vi "Sequencer.vi"() -> ()   [LabVIEW 2013]
uses:
  Tools/vars.ctl
  Tools/Line.ctl
  <vilib>/addons/h5labview2/file/H5Fmode.ctl
  Global.vi
  <vilib>/addons/h5labview2/base/lib_path.vi
  <vilib>/addons/h5labview2/base/H5Equery.vi
  <vilib>/addons/h5labview2/attrib/H5Awrite.llb/H5Awrite.xnode
  <vilib>/addons/h5labview2/file/H5F.lvlib
  <vilib>/addons/h5labview2/group/H5G.lvlib
  <vilib>/addons/h5labview2/attrib/H5A.lvlib
panel:
  in  "SQUID Comment":string
  out "uFiles":path[](array[path])
  in  "Save":bool=TRUE
  in  "stop":bool
  in  "Tab Control":enum32{"Run", "Settings", "Vars"}(tab)
  out "Status":string="<<Idle>>"
  out "Run List":string
  in  "Loops":i32=1 min=1
  in  "Run":bool
  in  "Run Tab":enum32{"Sequencer", "History"}(tab)
  in  "SEQ File":path caption="SEQ File (*.osq)"
  in  "Load List":bool
  out "VAR string":string[](array[string])
  out "Lines":i32
  out "History":cluster{"timestamp":timestamp, "File":path}[](array[cluster])=[{"timestamp"=timestamp(3546777743.6154723 s since 1904-01-01), "File"=path "C:/Users/Adam/Documents/oskar/Examples/example_chan.osq"}]
  out "RID":string="20160522_170223"
  in  "Abort":bool
  in  "Acquire (s)":i32=30
  out "Elapsed (s)":i32=30
  in  "Shuffle":bool
  out "HDF5 Save":path[](array[path])=[path "D:/Data/2016/05/22/20160522_170223/20160522_170223_raw.h5"]
  in  "Save Base":path[](array[path])=[path "D:/Data"]
  in  "Clear Run List Each Run":bool=TRUE
  out "error out":errorcluster
  out "hdf5":errorcluster
  in  "VARS":T1=[{"VAR"="CHAN", "Options"="A", "Val"="1", "Recieved"=FALSE, "Set"=FALSE}, {"VAR"="CHAN", "Options"="B", "Val"="2", "Recieved"=FALSE, "Set"=FALSE}, {"VAR"="CHAN", "Options"="C", "Val"="2", "Recieved"=FALSE, "Set"=FALSE}]
  in  "Override":bool
  out "All Set":bool
  out "Send":bool
  out "Recieved":bool
  in  "Pause":bool caption="Temporary wait before \nsetting next VAR array"
  # "Sequencer"
  # "name"
  # "options"
  # "value"
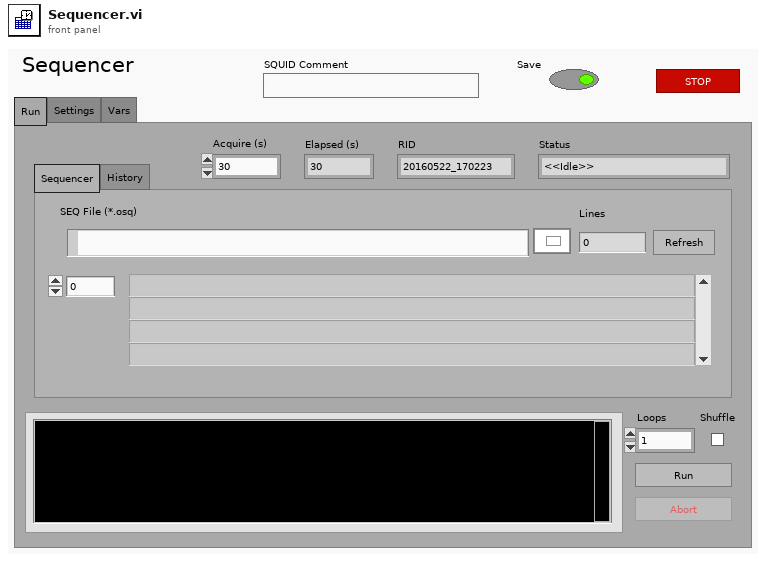
[diagram p1: front panel]
types:
  T1 = typedef "vars.ctl" = cluster{"VAR":string, "Options":string, "Val":string, "Recieved":bool, "Set":bool}[]
  T2 = cluster{"seconds since 1Jan1904":timestamp, string}
  T3 = enum32{"Invalid", "Standard", "Closed", "Hidden", "Minimized", "Maximized"}
  T4 = enum8{"Enabled", "Disabled", "Disabled and Grayed Out"}
  T5 = typedef "Line.ctl" = cluster{"Var Array":string[][], "Comment":string}
  T6 = typedef "H5F.lvlib/H5Fmode.ctl" = enum16{"read-only", "read-write", "overwrite", "create new", "open or create"}
  T7 = cluster{"VAR":string, "Options":string, "Val":string, "Recieved":bool, "Set":bool}
  T8 = cluster{"seconds since 1Jan1904":timestamp, "SEQ File":path}
  T9 = typedef "Semaphore RefNum" = refnum<k1>
  T10 = typedef "hid_t.ctl" = i32
  T11 = cluster{"VAR":string, "Options":string, "Val":string, "Recieved":bool, "Set":bool}[]
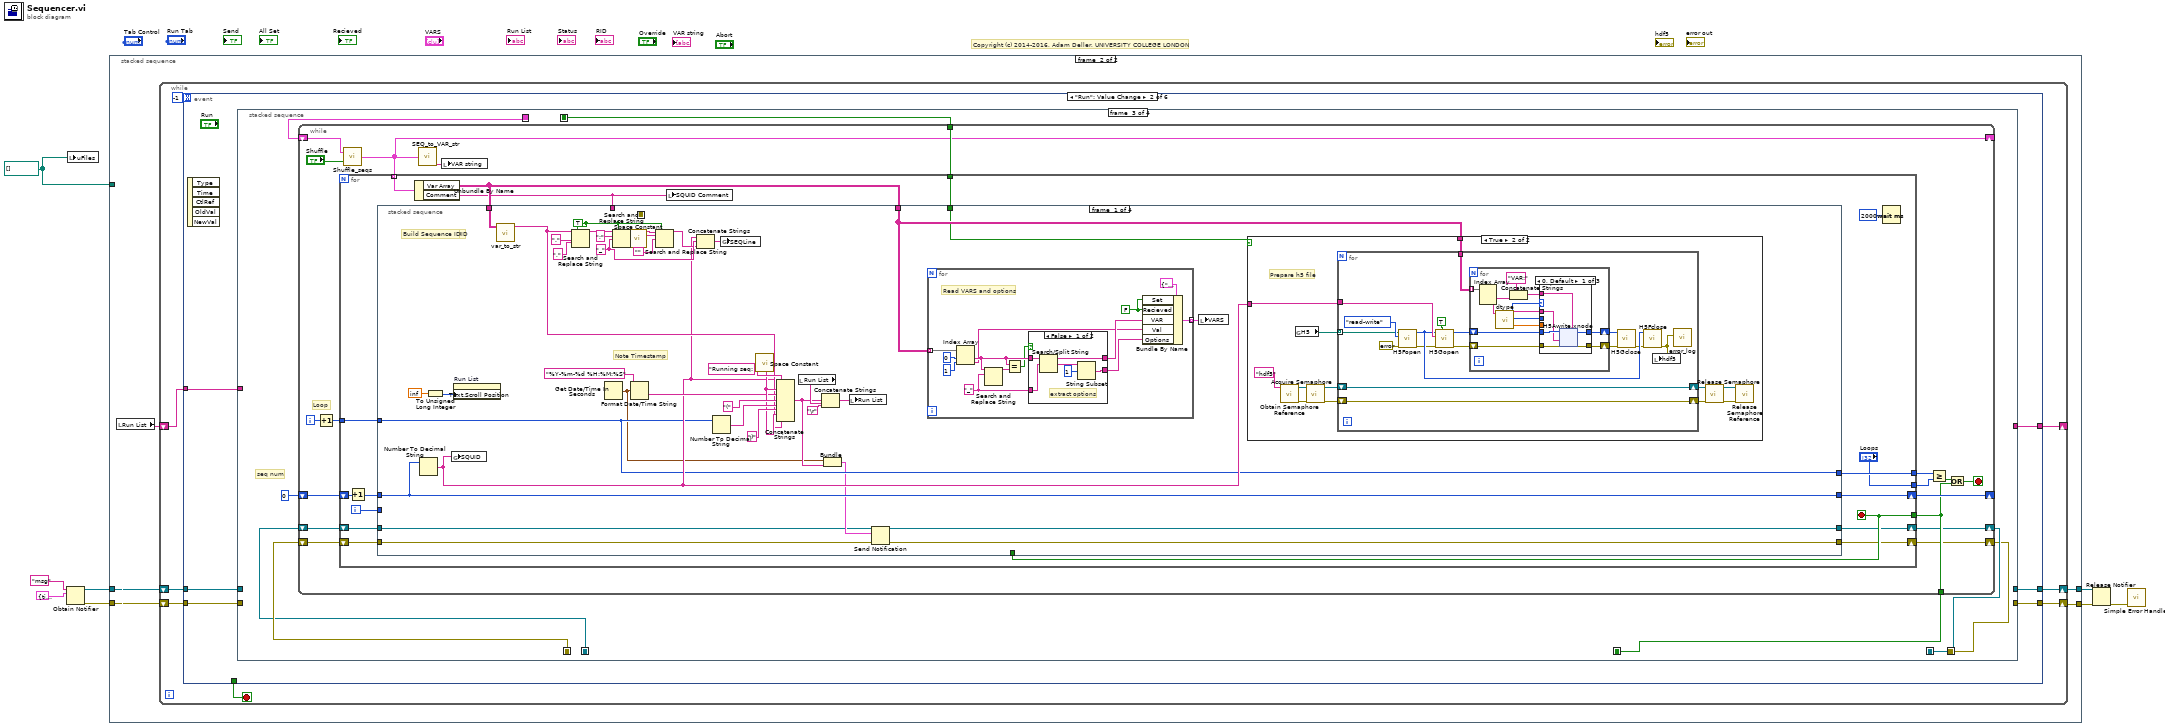
[diagram p0: block diagram]
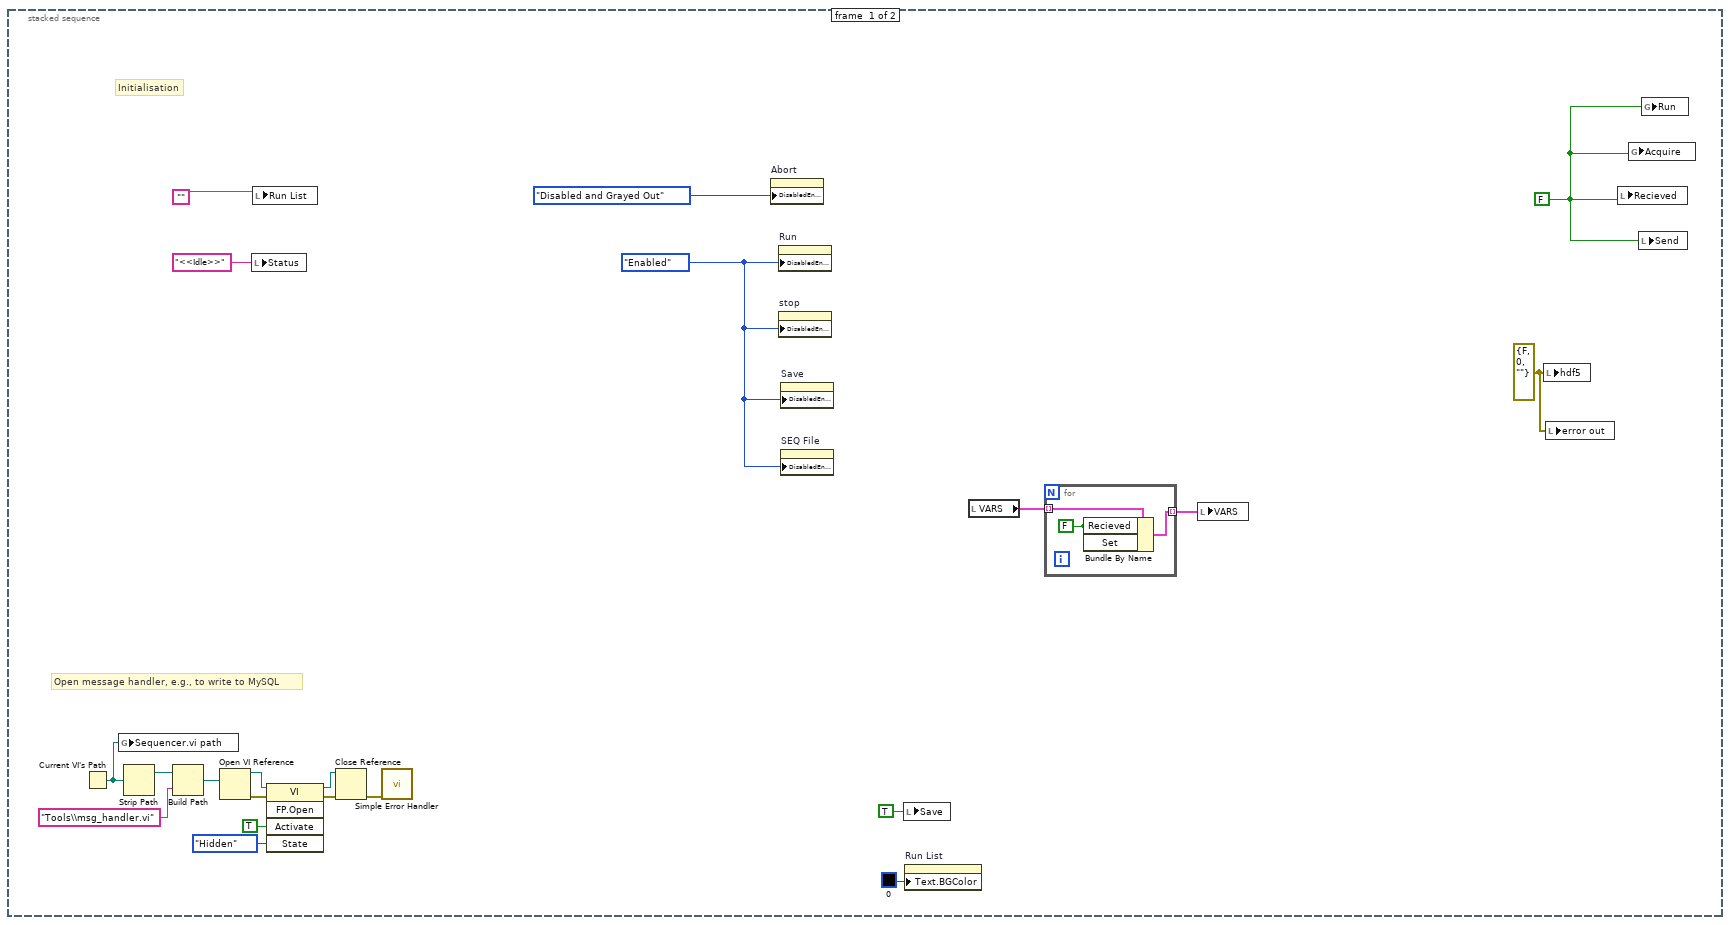
[diagram p2: hidden frame]
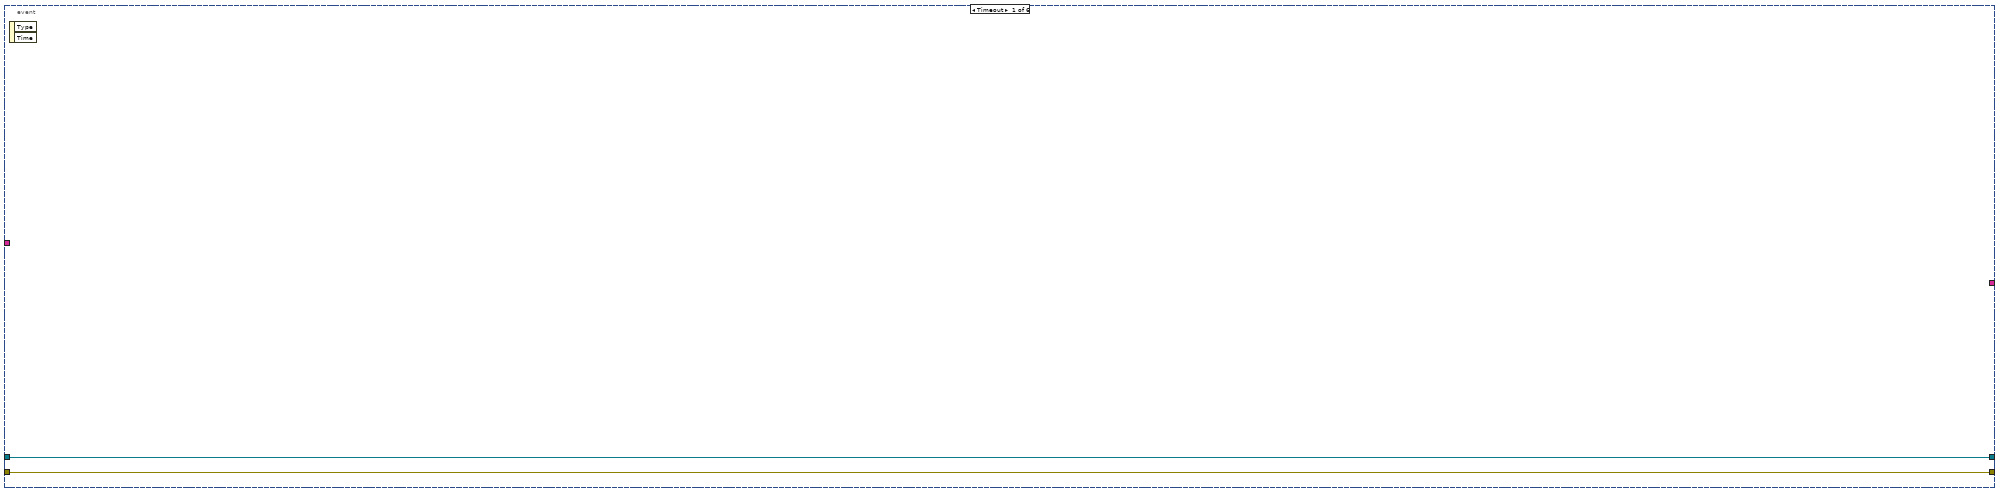
[diagram p3: hidden frame]
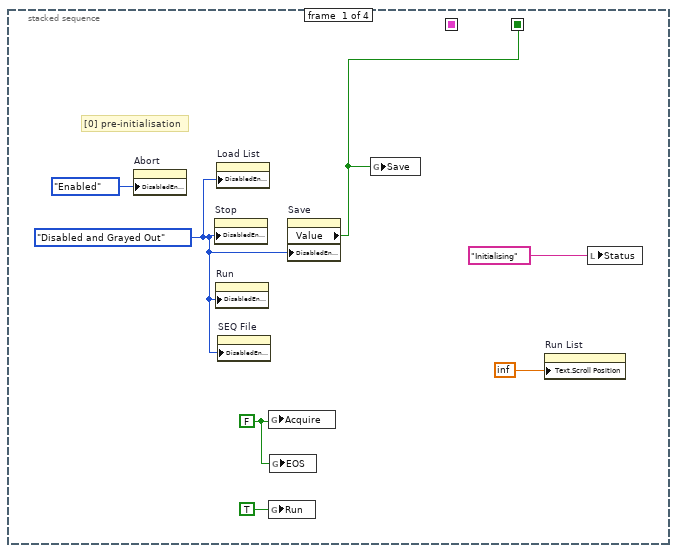
[diagram p4: hidden frame]
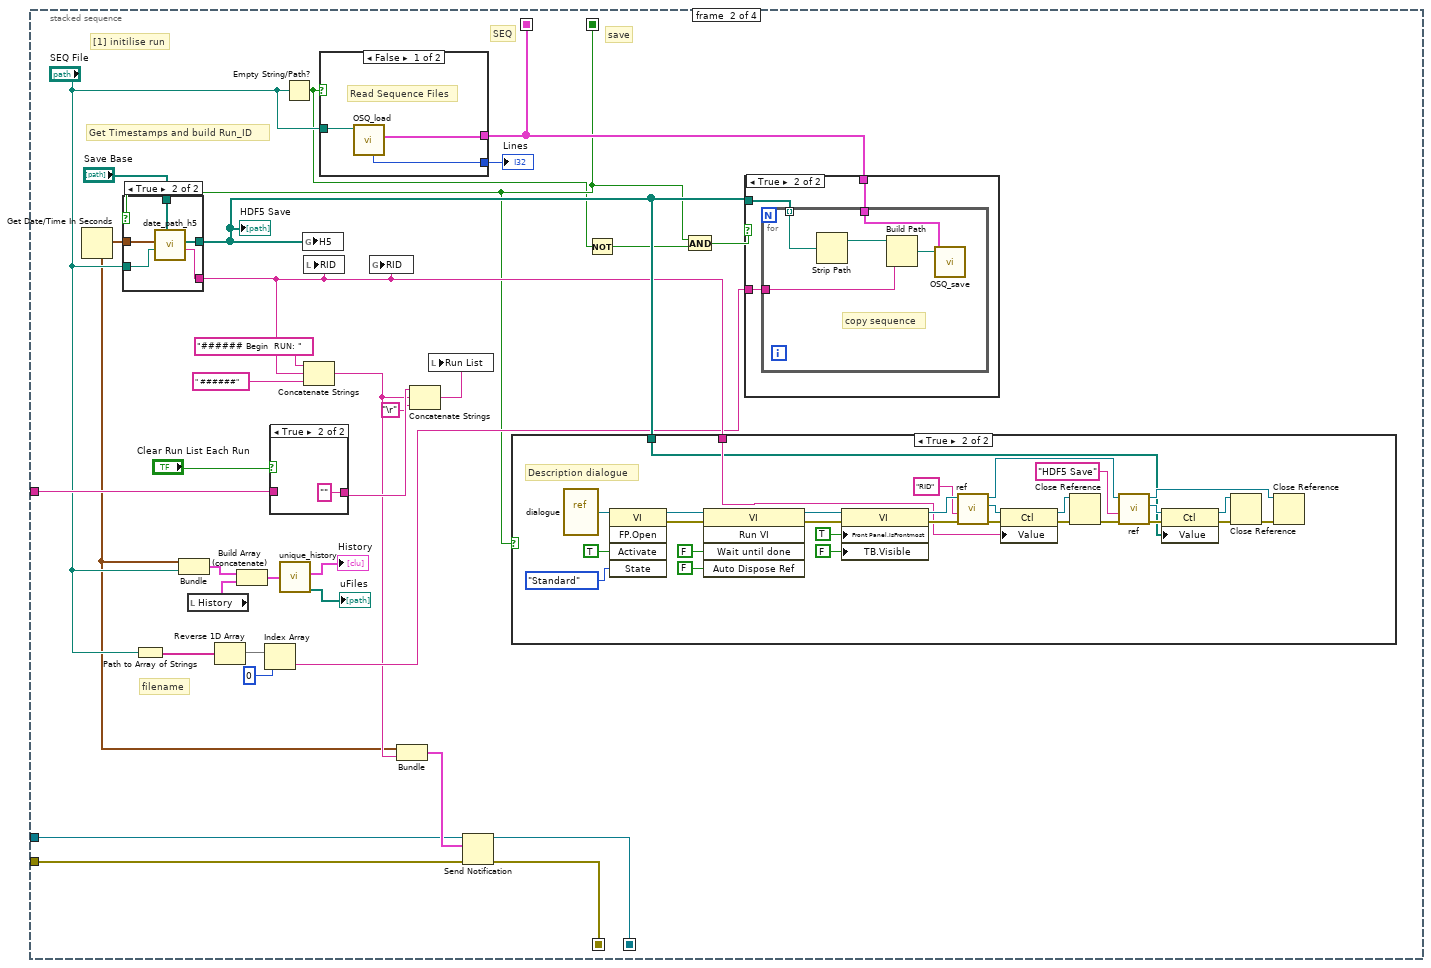
[diagram p5: hidden frame]
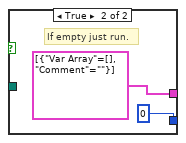
[diagram p7: hidden frame]
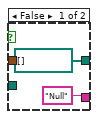
[diagram p8: hidden frame]
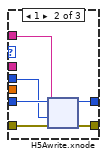
[diagram p12: hidden frame]
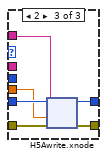
[diagram p13: hidden frame]
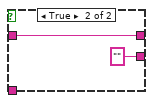
[diagram p14: hidden frame]
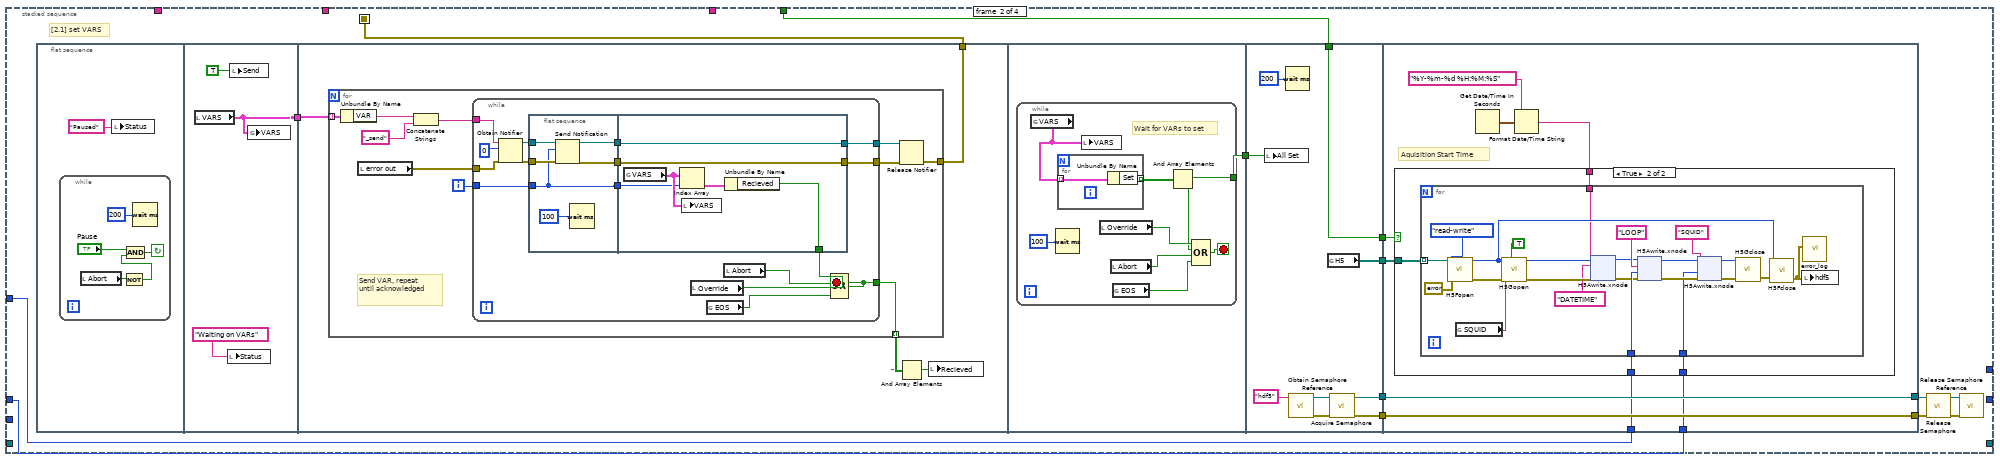
[diagram p15: hidden frame]
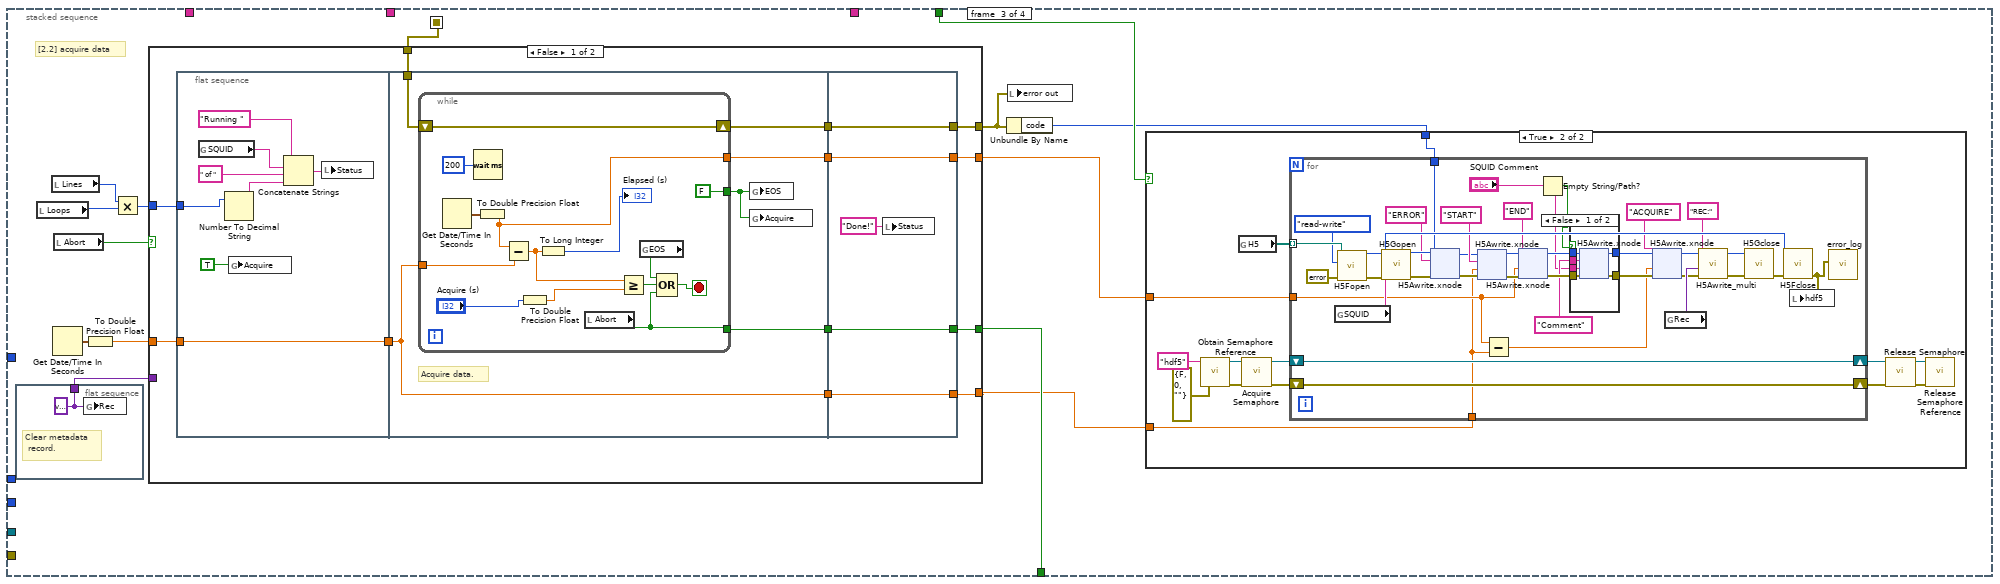
[diagram p17: hidden frame]
diagram:
  w8 = path[] [] ("uFiles")
  # "Copyright (c) 2014-2016, Adam Deller, UNIVERSITY COLLEGE LONDON"
  n1 = Obtain Notifier(name (unnamed)="msg", notification data type=T2 {"seconds since 1Jan1904"=timestamp(0 s since 1904-01-01), ""} ("output cluster")) -> (notifier out=w4:refnum<notifier>, error out=w5:errorcluster)  [unwired: 2 in, 1 out]
  n2 = local write "uFiles"(w8) -> ()
  n3 = stacked-sequence {
    tunnel: w8 -> [_ _]
    tunnel: w4 -> [_ w36]
    tunnel: w5 -> [_ w35]
    tunnel: [_ w34] -> w3
    tunnel: [_ w33] -> w2
    frame #0 {
      w20 = errorcluster {"status"=FALSE, "code"=0, "source"=""} ("hdf5")
      w22 = FALSE ("Send")
      w21 = T4."Enabled" ("Disabled")
      # "Open message handler, e.g., to write to MySQL"
      # "Initialisation"
      n4 = Current VI's Path() -> (path=w19:path)
      n5 = global write "Global.vi" "Sequencer.vi path"(w19) -> ()
      n6 = Strip Path(path=w19) -> (stripped path=w18:path)  [unwired: 1 out]
      n7 = Build Path(base path=w18, name or relative path="Tools\\msg_handler.vi") -> (appended path=w16:path)
      n8 = Open VI Reference(vi path=w16) -> (vi reference=w15:refnum<vi>, error out=w14:errorcluster)  [unwired: 5 in]
      n9 = local write "Status"("<<Idle>>" ("Status")) -> ()
      n10 = local write "Run List"("") -> ()
      n11 = invoke class="VI" method="FP.Open"(reference=w15, error in=w14, "Activate"=TRUE ("Activate?"), "State"=T3."Hidden") -> (reference out=w12:refnum<vi>, error out=w13:errorcluster)  [unwired: 1 in, 3 out]
      n12 = Close Reference(reference=w12, error in (no error)=w13) -> (error out=w9:errorcluster)
      n13 = call <vilib>:"Simple Error Handler.vi"("error in (no error)"=w9) -> ()  [unwired: 4 in, 5 out]
      n14 = property on="Abort" class="Bool (strict)"("DisabledEnum"=T4."Disabled and Grayed Out" ("Disabled")) -> ()  [unwired: 2 in, 2 out]
      n15 = property on="Run" class="Bool"("DisabledEnum"=w21) -> ()  [unwired: 2 in, 2 out]
      n16 = property on="stop" class="Bool"("DisabledEnum"=w21) -> ()  [unwired: 2 in, 2 out]
      n17 = property on="Save" class="Bool (strict)"("DisabledEnum"=w21) -> ()  [unwired: 2 in, 2 out]
      n18 = property on="SEQ File" class="Path"("DisabledEnum"=w21) -> ()  [unwired: 2 in, 2 out]
      n19 = local write "Save"(TRUE ("Save")) -> ()
      n20 = property on="Run List" class="Str"("Text.BGColor"=u32 0) -> ()  [unwired: 2 in, 2 out]
      n21 = local read "VARS"() -> (w27:T1)
      n22 = for {
        tunnel: [w32] -> w26 mode=indexing
        tunnel: w27 -> [w31] mode=indexing
        w30 = FALSE ("Set")
        n23 = Bundle By Name(cluster=w31, "Recieved"=w30, "Set"=w30) -> (w32:T7)
      }
      n24 = local write "VARS"(w26) -> ()
      n25 = local write "hdf5"(w20) -> ()
      n26 = local write "error out"(w20) -> ()
      n27 = local write "Recieved"(w22) -> ()
      n28 = global write "Global.vi" "Acquire"(w22) -> ()
      n29 = local write "Send"(w22) -> ()
      n30 = global write "Global.vi" "Run"(w22) -> ()
    }
    frame #1 {
      n31 = local read "Run List"() -> (w37:string)
      n32 = while {
        shift-right: [w42] -> _
        shift-left: w37 -> [w43]
        shift-right: [w39] -> w33
        shift-left: w36 -> [w41]
        shift-right: [w38] -> w34
        shift-left: w35 -> [w40]
        stop <- w45 stop-if-true
        n33 = event shown="[1] \"Run\": Value Change" {
          selector: _ -> [_ _ _ _ _ _]
          dyn-events: _ -> [_ _ _ _ _ _]
          timeout: -1 -> [_ _ _ _ _ _]
          tunnel: [_ _ _ _ _ "stop"] -> w45
          tunnel: w43 -> [_ w53 _ _ _ _]
          tunnel: [_ w52 _ _ _ _] -> w42
          tunnel: w41 -> [w47 w51 w779 w791 w797 w809]
          tunnel: w40 -> [w46 w50 w778 w790 w796 w808]
          tunnel: [w47 w49 w779 w791 w797 w809] -> w39
          tunnel: [w46 w48 w778 w790 w796 w808] -> w38
          event Timeout {
            n34 = event-data() -> ()  [unwired: 1 in, 2 out]
          }
          event "Run": Value Change {
            n35 = event-data() -> ()  [unwired: 1 in, 5 out]
            n36 = stacked-sequence {
              seq-local: [_ _ w152 _] -> [_ _ _ w760]
              seq-local: [w58 _ _ _] -> [_ w71 w151 _]
              seq-local: [_ w77 _ _] -> [_ _ w149 _]
              seq-local: [_ w62 _ _] -> [_ _ w148 _]
              seq-local: [_ w61 _ _] -> [_ _ w147 _]
              seq-local: [_ _ w146 _] -> [_ _ _ w758]
              seq-local: [_ _ w145 _] -> [_ _ _ w759]
              tunnel: w53 -> [_ w93 _ _]
              tunnel: [_ _ _ w761] -> w52
              tunnel: w51 -> [_ w63 _ _]
              tunnel: w50 -> [_ w65 _ _]
              tunnel: [_ _ _ w754] -> w49
              tunnel: [_ _ _ w753] -> w48
              frame #0 {
                w56 = FALSE ("Save")
                w55 = T4."Disabled and Grayed Out" ("Disabled")
                # "[0] pre-initialisation"
                n37 = property on="Abort" class="Bool (strict)"("DisabledEnum"=T4."Enabled" ("Disabled")) -> ()  [unwired: 2 in, 2 out]
                n38 = property on="Stop" class="Bool"("DisabledEnum"=w55) -> ()  [unwired: 2 in, 2 out]
                n39 = property on="Run" class="Bool"("DisabledEnum"=w55) -> ()  [unwired: 2 in, 2 out]
                n40 = property on="Load List" class="Bool"("DisabledEnum"=w55) -> ()  [unwired: 2 in, 2 out]
                n41 = property on="SEQ File" class="Path"("DisabledEnum"=w55) -> ()  [unwired: 2 in, 2 out]
                n42 = global write "Global.vi" "Acquire"(w56) -> ()
                n43 = global write "Global.vi" "Run"(TRUE ("Run on now")) -> ()
                n44 = global write "Global.vi" "EOS"(w56) -> ()
                n45 = property on="Save" class="Bool (strict)"("DisabledEnum"=w55) -> ("Value"=w58:bool)  [unwired: 2 in, 2 out]
                n46 = global write "Global.vi" "Save"(w58) -> ()
                n47 = property on="Run List" class="Str"("Text.Scroll Position"=inf) -> ()  [unwired: 2 in, 2 out]
                n48 = local write "Status"("Initialising" ("Status")) -> ()
              }
              frame #1 {
                # "filename"
                # "save"
                # "SEQ"
                # "[1] initilise run"
                # "Get Timestamps and build Run_ID"
                n49 = Get Date/Time In Seconds() -> (seconds since 1Jan1904=w66:timestamp)
                n50 = case shown="True" w71 {
                  tunnel: w66 -> [_ w134]
                  tunnel: ["Null" ("RID") w133] -> w78
                  tunnel: "Save Base" -> [_ w132]
                  tunnel: [path[] [] ("Paths") w131] -> w79
                  tunnel: "SEQ File" -> [_ w130]
                  frame False {
                  }
                  frame True {
                    n51 = call "date_path_h5.vi"("Bases"=w132, "SEQ File"=w130, "time stamp"=w134) -> ("RID"=w133:string, "H5"=w131:path[])  [unwired: 7 in]
                  }
                }
                "HDF5 Save" <- w79
                n52 = Path to Array of Strings(0:"SEQ File") -> (2:w75:string[])  [unwired: 1 out]
                n53 = Bundle("seconds since 1Jan1904"=w66, "SEQ File"="SEQ File") -> (w81:T8)  [unwired: 1 in]
                n54 = local read "History"() -> (w85:cluster{"timestamp":timestamp, "File":path}[])
                n55 = Reverse 1D Array(array=w75) -> (reversed array=w74:string[])
                n56 = Build Array (concatenate)(w81, w85) -> (w84:cluster{"timestamp":timestamp, "File":path}[])
                n57 = Index Array(array=w74, index=0) -> (element=w72:string)
                n58 = case shown="True" "Clear Run List Each Run" {
                  tunnel: w93 -> [w143 _]
                  tunnel: [w143 "" ("Log")] -> w91
                  frame False {
                  }
                  frame True {
                  }
                }
                n59 = call "unique_history.vi"("History In"=w84) -> ("uFiles"=→"uFiles":path[], "History Out"=→"History":cluster{"Time Stamp":timestamp, "Path":path}[])  [unwired: 9 in]
                n60 = Empty String/Path?(string/path="SEQ File") -> (empty?=w70:bool)
                n61 = global write "Global.vi" "H5"(w79) -> ()
                n62 = local write "RID"(w78) -> ()
                n63 = Concatenate Strings("###### Begin  RUN: " ("string"), w78, " ######" ("string")) -> (w67:string)
                n64 = case shown="False" w70 {
                  tunnel: "SEQ File" -> [w124 _]
                  tunnel: [w125 0 ("Lines")] -> w80
                  tunnel: [w123 T5[] [{"Var Array"=[], "Comment"=""}] ("SEQs")] -> w77
                  frame False {
                    # "Read Sequence Files"
                    n65 = call "OSQ_load.vi"("Open"=w124) -> ("SEQs"=w123:T5[], "Lines"=w125:i32)  [unwired: 7 in, 2 out]
                  }
                  frame True {
                    # "If empty just run."
                  }
                }
                "Lines" <- w80
                n66 = global write "Global.vi" "RID"(w78) -> ()
                n67 = Bundle("seconds since 1Jan1904"=w66, w67) -> (w64:T2)  [unwired: 1 in]
                n68 = Concatenate Strings(w91, w67, "\r") -> (w90:string)
                n69 = local write "Run List"(w90) -> ()
                n70 = Send Notification(notification=w64, notifier=w63, error in (no error)=w65) -> (notifier out=w61:refnum<notifier>, error out=w62:errorcluster)
                n71 = case shown="True" w71 {
                  tunnel: w79 -> [_ w94]
                  tunnel: w78 -> [_ w95]
                  frame False {
                  }
                  frame True {
                    # "Description dialogue"
                    n72 = vi-ref "dialogue.vi"() -> (w121:refnum<vi>)
                    n73 = invoke class="VI" method="FP.Open"(reference=w121, "Activate"=TRUE ("Activate?"), "State"=T3."Standard") -> (reference out=w102:refnum<vi>, error out=w99:errorcluster)  [unwired: 2 in, 3 out]
                    n74 = invoke class="VI" method="Run VI"(reference=w102, error in=w99, "Wait until done"=FALSE ("Wait Until Done"), "Auto Dispose Ref"=FALSE ("Auto Dispose Reference")) -> (reference out=w101:refnum<vi>, error out=w100:errorcluster)  [unwired: 1 in, 3 out]
                    n75 = property class="VI"(reference=w101, error in=w100, "Front Panel.IsFrontmost"=TRUE ("Front Panel Window:Is Frontmost"), "TB.Visible"=FALSE ("Tool Bar:Visible")) -> (reference out=w118:refnum<vi>, error out=w117:errorcluster)
                    n76 = call "ref.vi"("error in (no error)"=w117, "Name"="RID", "VI reference"=w118) -> ("error out"=w111:errorcluster, "Ctrl reference out"=w112:refnum<vi>, "VI reference out"=w115:refnum<vi>)  [unwired: 5 in, 1 out]
                    n77 = property class="Ctl"(reference=w112, error in=w111, "Value"=w95) -> (reference out=w109:refnum<vi>, error out=w110:errorcluster)
                    n78 = Close Reference(reference=w109, error in (no error)=w110) -> (error out=w108:errorcluster)
                    n79 = call "ref.vi"("error in (no error)"=w108, "Name"="HDF5 Save", "VI reference"=w115) -> ("error out"=w107:errorcluster, "Ctrl reference out"=w103:refnum<vi>, "VI reference out"=w113:refnum<vi>)  [unwired: 5 in, 1 out]
                    n80 = property class="Ctl"(reference=w103, error in=w107, "Value"=w94) -> (reference out=w104:refnum<vi>, error out=w106:errorcluster)
                    n81 = Close Reference(reference=w104, error in (no error)=w106) -> (error out=w105:errorcluster)
                    n82 = Close Reference(reference=w113, error in (no error)=w105) -> ()  [unwired: 1 out]
                  }
                }
                n83 = Not(x=w70) -> (.not. x?=w69:bool)
                n84 = And(x=w71, y=w69) -> (x .and. y?=w68:bool)
                n85 = case shown="True" w68 {
                  tunnel: w72 -> [_ w137]
                  tunnel: w79 -> [_ w136]
                  tunnel: w77 -> [_ w135]
                  frame False {
                  }
                  frame True {
                    n86 = for {
                      tunnel: w137 -> [w138]
                      tunnel: w136 -> [w140] mode=indexing
                      tunnel: w135 -> [w141]
                      # "copy sequence"
                      n87 = Strip Path(path=w140) -> (stripped path=w139:path)  [unwired: 1 out]
                      n88 = Build Path(base path=w139, name or relative path=w138) -> (appended path=w142:path)
                      n89 = call "OSQ_save.vi"("SEQs"=w141, "Save"=w142) -> ()  [unwired: 8 in, 2 out]
                    }
                  }
                }
              }
              frame #2 {
                # "seq num"
                n90 = while {
                  tunnel: [w157] -> w152
                  tunnel: w151 -> [w170]
                  shift-right: [w168] -> _
                  shift-left: 0 -> [w169]
                  shift-right: [w162] -> _
                  shift-left: w149 -> [w164]
                  shift-right: [w153] -> w146
                  shift-left: w147 -> [w156]
                  shift-right: [w154] -> w145
                  shift-left: w148 -> [w155]
                  i -> [w166]
                  stop <- w159 stop-if-true
                  # "Loop"
                  n91 = Increment(x=w166) -> (x+1=w167:i32)
                  n92 = call "Shuffle_seqs.vi"("Shuffle"="Shuffle", "Array IN"=w164) -> ("Array OUT"=w162:T5[])
                  n93 = for {
                    tunnel: [w175] -> w157
                    tunnel: w170 -> [w187]
                    shift-right: [w185] -> w168
                    shift-left: w169 -> [w181]
                    tunnel: w162 -> [w183] mode=indexing
                    tunnel: w167 -> [w180]
                    tunnel: [w177] -> w161
                    tunnel: ["Loops"] -> w158
                    shift-right: [w172] -> w153
                    shift-left: w156 -> [w174]
                    shift-right: [w171] -> w154
                    shift-left: w155 -> [w173]
                    i -> [w184]
                    stop <- w175 stop-if-true
                    n94 = Increment(x=w181) -> (x+1=w182:i32)
                    n95 = Unbundle By Name(w183) -> ("Var Array"=w179:string[][], "Comment"=w178:string)
                    n96 = stacked-sequence {
                      seq-local: [_ w372 _ _] -> [_ _ w548 _]
                      tunnel: [_ _ w547 _] -> w175
                      tunnel: w187 -> [w198 w363 w545 _]
                      tunnel: [w215 _ _ _] -> w185
                      tunnel: w184 -> [_ _ _ _]
                      tunnel: w179 -> [w199 _ _ _]
                      tunnel: w182 -> [w215 w360 _ _]
                      tunnel: w180 -> [w196 w361 _ _]
                      tunnel: w178 -> [_ _ _ _]
                      tunnel: w179 -> [w201 _ _ _]
                      tunnel: [w196 _ _ _] -> w177
                      tunnel: w174 -> [w191 _ _ _]
                      tunnel: w173 -> [w190 _ _ _]
                      tunnel: [w189 _ _ _] -> w172
                      tunnel: [w188 _ _ _] -> w171
                      frame #0 {
                        w207 = TRUE ("replace all? (F)")
                        w206 = "_" ("replace string (\"\")")
                        # "[2.0] initialise SQUID"
                        # "Note Timestamp"
                        # "Build Sequence ID"
                        n97 = Number To Decimal String(number=w215) -> (decimal integer string=w197:string)  [unwired: 1 in]
                        n98 = To Unsigned Long Integer(number=inf) -> (unsigned 32bit integer=w202:u32)
                        n99 = global write "Global.vi" "SQUID"(w197) -> ()
                        n100 = property on="Run List" class="Str"("Text.Scroll Position"=w202) -> ()  [unwired: 2 in, 2 out]
                        n101 = call "var_to_str.vi"("Var Array"=w201) -> ("VAR string"=w200:string)  [unwired: 10 in]
                        n102 = Search and Replace String(replace all?=w207, input string=w200, search string=".", replace string="," ("replace string (\"\")")) -> (result string=w208:string)  [unwired: 4 in, 3 out]
                        n103 = Get Date/Time In Seconds() -> (seconds since 1Jan1904=w193:timestamp)
                        n104 = Search and Replace String(replace all?=w207, input string=w208, search string=";", replace string=w206) -> (result string=w211:string)  [unwired: 4 in, 3 out]
                        n105 = call <vilib>:"Space Constant.vi"() -> ("String"=w213:string)
                        n106 = Format Date/Time String(time format string (%c)="%Y-%m-%d %H:%M:%S", seconds (now)=w193) -> (date/time string=w219:string)  [unwired: 1 in]
                        n107 = Search and Replace String(replace all?=w207, input string=w211, search string=w213, replace string="") -> (result string=w205:string)  [unwired: 4 in, 3 out]
                        n108 = Concatenate Strings(w197, w206, w205) -> (w204:string)
                        n109 = Number To Decimal String(number=w196) -> (decimal integer string=w222:string)  [unwired: 1 in]
                        n110 = global write "Global.vi" "SEQLine"(w204) -> ()
                        n111 = call <vilib>:"Space Constant.vi"() -> ("String"=w220:string)
                        n112 = Concatenate Strings(w219, w220, "Running seq: " ("string"), w197, "(" ("string"), w222, ")" ("string"), w220, w200) -> (w194:string)
                        n113 = local read "Run List"() -> (w218:string)
                        n114 = Concatenate Strings(w218, w194, "\r") -> (w217:string)
                        n115 = Bundle("seconds since 1Jan1904"=w193, w194) -> (w192:T2)  [unwired: 1 in]
                        n116 = local write "Run List"(w217) -> ()
                        n117 = Send Notification(notification=w192, notifier=w191, error in (no error)=w190) -> (notifier out=w189:refnum<notifier>, error out=w188:errorcluster)
                        n118 = for {
                          tunnel: w199 -> [w349] mode=indexing
                          tunnel: [w348] -> w195 mode=indexing
                          w341 = "_" ("search string/char (-)")
                          w346 = FALSE ("Set")
                          # "Read VARS and options"
                          n119 = Index Array(array=w349, index #1=0 ("index"), index #2=1 ("index")) -> (element #1=w342:string, element #2=w339:string)
                          n120 = Search and Replace String(input string=w342, search string=w341) -> (result string=w343:string)  [unwired: 6 in, 3 out]
                          n121 = Equal?(x=w342, y=w343) -> (x = y?=w340:bool)
                          n122 = case shown="False" w340 {
                            tunnel: [w357 w358] -> w345
                            tunnel: [w354 "" ("String")] -> w344
                            tunnel: w342 -> [w353 w358]
                            tunnel: w341 -> [w352 _]
                            frame False {
                              # "extract options"
                              n123 = Search/Split String(string=w353, search string/char (-)=w352) -> (substring before match=w357:string, match + rest of string=w356:string)  [unwired: 1 in, 1 out]
                              n124 = String Subset(string=w356, offset (0)=1) -> (substring=w354:string)  [unwired: 1 in]
                            }
                            frame True {
                            }
                          }
                          n125 = Bundle By Name(cluster=T7 {"VAR"="", "Options"="", "Val"="", "Recieved"=FALSE, "Set"=FALSE} ("VARS 2"), "Set"=w346, "Recieved"=w346, "VAR"=w345, "Val"=w339, "Options"=w344) -> (w348:T7)
                        }
                        n126 = local write "VARS"(w195) -> ()
                        n127 = case shown="True" w198 {
                          tunnel: w197 -> [_ w236]
                          tunnel: w199 -> [_ w235]
                          frame False {
                          }
                          frame True {
                            # "Prepare h5 file"
                            n128 = call <vilib>:"Obtain Semaphore Reference.vi"("name (unnamed)"="hdf5") -> ("error out"=w233:errorcluster, "semaphore"=w234:T9)  [unwired: 4 in, 1 out]
                            n129 = global read "Global.vi" "H5"() -> (w237:path[])
                            n130 = call <vilib>:"Acquire Semaphore.vi"("error in (no error)"=w233, "semaphore"=w234) -> ("error out"=w228:errorcluster, "semaphore out"=w229:T9)  [unwired: 3 in, 1 out]
                            n131 = for {
                              tunnel: w237 -> [w252] mode=indexing
                              tunnel: w236 -> [w251]
                              tunnel: w235 -> [w245]
                              shift-right: [w243] -> w227
                              shift-left: w229 -> [w243]
                              shift-right: [w244] -> w226
                              shift-left: w228 -> [w244]
                              n132 = call <vilib>:"H5Fopen.vi"("error in (no error)"=errorcluster {"status"=FALSE, "code"=0, "source"=""} ("error out"), "mode (read-only)"=H5Fmode."read-write", "path"=w252) -> ("error out"=w242:errorcluster, "ref out"=w249:T10)  [unwired: 7 in]
                              n133 = call <vilib>:"H5Gopen.vi"("create? (F)"=TRUE, "error in (no error)"=w242, "name"=w251, "ref in"=w249) -> ("error out"=w241:errorcluster, "group out"=w240:T10)  [unwired: 6 in]
                              n134 = for {
                                tunnel: w245 -> [w264] mode=indexing
                                shift-right: [w266] -> w247
                                shift-left: w240 -> [w259]
                                shift-right: [w265] -> w246
                                shift-left: w241 -> [w258]
                                n135 = Index Array(array=w264) -> (element #1=w263:string, element #2=w260:string)  [unwired: 2 in]
                                n136 = call "dtype.vi"("String"=w260) -> ("DBL"=w254:dbl, "I32"=w255:i32, "String out"=w256:string, "dtype (0:str, 1:i32, 2:f64)"=w257:u32)  [unwired: 7 in]
                                n137 = Concatenate Strings("VAR:" ("string"), w263) -> (w261:string)
                                n138 = case shown="0, Default" w257 {
                                tunnel: [w270 w296 w318] -> w266
                                tunnel: [w271 w295 w319] -> w265
                                tunnel: w261 -> [w268 w294 w316]
                                tunnel: w259 -> [w269 w293 w317]
                                tunnel: w258 -> [w272 w292 w320]
                                tunnel: w256 -> [w267 _ _]
                                tunnel: w255 -> [_ w291 _]
                                tunnel: w254 -> [_ _ w315]
                                frame 0, Default {
                                n139 = xnode "H5Awrite.xnode"("error in (no error)"=w272, "data"=w267, "attrib name"=w268, "ref in"=w269) -> ("error out"=w271:errorcluster, "ref out"=w270:i32)  [unwired: 3 in, 1 out]
                                }
                                frame 1 {
                                n140 = xnode "H5Awrite.xnode"("error in (no error)"=w292, "data"=w291, "attrib name"=w294, "ref in"=w293) -> ("error out"=w295:errorcluster, "ref out"=w296:i32)  [unwired: 3 in, 1 out]
                                }
                                frame 2 {
                                n141 = xnode "H5Awrite.xnode"("error in (no error)"=w320, "data"=w315, "attrib name"=w316, "ref in"=w317) -> ("error out"=w319:errorcluster, "ref out"=w318:i32)  [unwired: 3 in, 1 out]
                                }
                                }
                              }
                              n142 = call <vilib>:"H5Gclose.vi"("error in (no error)"=w246, "group in"=w247) -> ("error out"=w248:errorcluster)  [unwired: 9 in]
                              n143 = call <vilib>:"H5Fclose.vi"("error in (no error)"=w248, "ref"=w249) -> ("error out"=w238:errorcluster)  [unwired: 9 in]
                              n144 = local write "hdf5"(w238) -> ()
                              n145 = call "error_log.vi"("error"=w238) -> ()  [unwired: 10 in]
                            }
                            n146 = call <vilib>:"Release Semaphore.vi"("error in (no error)"=w226, "semaphore"=w227) -> ("error out"=w231:errorcluster, "semaphore out"=w230:T9)  [unwired: 4 in]
                            n147 = call <vilib>:"Release Semaphore Reference.vi"("error in (no error)"=w231, "semaphore"=w230) -> ()  [unwired: 8 in, 2 out]
                          }
                        }
                      }
                      frame #1 {
                        # "[2.1] set VARS"
                        n148 = flat-sequence {
                          tunnel: [w382] -> w373
                          tunnel: w373 -> [w386]
                          tunnel: [w383] -> w372
                          tunnel: [w425] -> w371
                          tunnel: w371 -> [w443]
                          tunnel: [w439] -> w367
                          tunnel: [w438] -> w365
                          tunnel: [w437] -> w364
                          tunnel: w363 -> [w437]
                          tunnel: [w436] -> w362
                          tunnel: [w452] -> w368
                          tunnel: w367 -> [w452]
                          tunnel: [w451] -> w366
                          tunnel: w365 -> [w451]
                          tunnel: w364 -> [w450]
                          tunnel: w362 -> [w449]
                          tunnel: w361 -> [w446]
                          tunnel: w360 -> [w445]
                          frame #0 {
                            n149 = while {
                              stop <- w377 continue-if-true
                              n150 = local read "Abort"() -> (w378:bool)
                              n151 = Not(x=w378) -> (.not. x?=w376:bool)
                              n152 = And(x="Pause", y=w376) -> (x .and. y?=w377:bool)
                              n153 = Wait (ms)(milliseconds to wait=u32 200) -> ()  [unwired: 1 out]
                            }
                            n154 = local write "Status"("Paused" ("Status")) -> ()
                          }
                          frame #1 {
                            n155 = local read "VARS"() -> (w382:T1)
                            n156 = local write "Status"("Waiting on VARs" ("Status")) -> ()
                            n157 = local write "Send"(TRUE ("Send")) -> ()
                            n158 = global write "Global.vi" "VARS"(w382) -> ()
                          }
                          frame #2 {
                            n159 = for {
                              tunnel: w386 -> [w396] mode=indexing
                              tunnel: [w392] -> w385 mode=indexing
                              tunnel: [w389] -> w383
                              i -> [w393]
                              # "Send VAR, repeat until acknowledged"
                              n160 = Unbundle By Name(w396) -> ("VAR"=w394:string)
                              n161 = local read "error out"() -> (w387:errorcluster)
                              n162 = Concatenate Strings(w394, "_send") -> (w388:string)
                              n163 = while {
                                tunnel: w393 -> [w408]
                                tunnel: [w403] -> w392
                                tunnel: [w411] -> w391
                                tunnel: [w410] -> w390
                                tunnel: w388 -> [w401]
                                tunnel: w387 -> [w397]
                                stop <- w403 stop-if-true
                                n164 = Obtain Notifier(name (unnamed)=w401, notification data type=0, error in (no error)=w397) -> (notifier out=w399:refnum<notifier>, error out=w400:errorcluster)  [unwired: 1 in, 1 out]
                                n165 = flat-sequence {
                                tunnel: w399 -> [w417]
                                tunnel: w400 -> [w418]
                                tunnel: [w416] -> w412
                                tunnel: [w415] -> w409
                                tunnel: w408 -> [w413]
                                tunnel: [w413] -> w407
                                tunnel: [w421] -> w404
                                tunnel: [w423] -> w411
                                tunnel: w412 -> [w423]
                                tunnel: [w422] -> w410
                                tunnel: w409 -> [w422]
                                tunnel: w407 -> [w419]
                                frame #0 {
                                n166 = Send Notification(notification=w413, notifier=w417, error in (no error)=w418) -> (notifier out=w416:refnum<notifier>, error out=w415:errorcluster)
                                n167 = Wait (ms)(milliseconds to wait=u32 100) -> ()  [unwired: 1 out]
                                }
                                frame #1 {
                                n168 = global read "Global.vi" "VARS"() -> (w420:T11)
                                n169 = Index Array(array=w420, index=w419) -> (element=w424:T7)
                                n170 = local write "VARS"(w420) -> ()
                                n171 = Unbundle By Name(w424) -> ("Recieved"=w421:bool)
                                }
                                }
                                n172 = local read "Override"() -> (w405:bool)
                                n173 = global read "Global.vi" "EOS"() -> (w398:bool)
                                n174 = local read "Abort"() -> (w406:bool)
                                n175 = Compound Arithmetic op=OR(w404, w406, w405, w398) -> (w403:bool)
                              }
                              n176 = Release Notifier(notifier=w391, error in (no error)=w390) -> (error out=w389:errorcluster)  [unwired: 1 in, 2 out]
                            }
                            n177 = And Array Elements(Boolean array=w385) -> (logical AND=w384:bool)
                            n178 = local write "Recieved"(w384) -> ()
                          }
                          frame #3 {
                            n179 = while {
                              tunnel: [w428] -> w425
                              stop <- w427 stop-if-true
                              # "Wait for VARs to set"
                              n180 = global read "Global.vi" "VARS"() -> (w431:T11)
                              n181 = Wait (ms)(milliseconds to wait=u32 100) -> ()  [unwired: 1 out]
                              n182 = for {
                                tunnel: w431 -> [w435] mode=indexing
                                tunnel: [w434] -> w433 mode=indexing
                                n183 = Unbundle By Name(w435) -> ("Set"=w434:bool)
                              }
                              n184 = local write "VARS"(w431) -> ()
                              n185 = local read "Override"() -> (w430:bool)
                              n186 = local read "Abort"() -> (w429:bool)
                              n187 = global read "Global.vi" "EOS"() -> (w426:bool)
                              n188 = And Array Elements(Boolean array=w433) -> (logical AND=w428:bool)
                              n189 = Compound Arithmetic op=OR(w430, w428, w429, w426) -> (w427:bool)
                            }
                          }
                          frame #4 {
                            n190 = local write "All Set"(w443) -> ()
                            n191 = Wait (ms)(milliseconds to wait=u32 200) -> ()  [unwired: 1 out]
                            n192 = call <vilib>:"Obtain Semaphore Reference.vi"("name (unnamed)"="hdf5") -> ("error out"=w441:errorcluster, "semaphore"=w440:T9)  [unwired: 4 in, 1 out]
                            n193 = global read "Global.vi" "H5"() -> (w436:path[])
                            n194 = call <vilib>:"Acquire Semaphore.vi"("error in (no error)"=w441, "semaphore"=w440) -> ("error out"=w438:errorcluster, "semaphore out"=w439:T9)  [unwired: 3 in, 1 out]
                          }
                          frame #5 {
                            # "Aquisition Start Time"
                            n195 = Get Date/Time In Seconds() -> (seconds since 1Jan1904=w447:timestamp)
                            n196 = Format Date/Time String(time format string (%c)="%Y-%m-%d %H:%M:%S", seconds (now)=w447) -> (date/time string=w448:string)  [unwired: 1 in]
                            n197 = case shown="True" w450 {
                              tunnel: w449 -> [_ w457]
                              tunnel: w448 -> [_ w456]
                              tunnel: w446 -> [_ w455]
                              tunnel: w445 -> [_ w454]
                              frame False {
                              }
                              frame True {
                                n198 = for {
                                tunnel: w457 -> [w479] mode=indexing
                                tunnel: w456 -> [w474]
                                tunnel: w455 -> [w468]
                                tunnel: w454 -> [w462]
                                n199 = call <vilib>:"H5Fopen.vi"("error in (no error)"=errorcluster {"status"=FALSE, "code"=0, "source"=""} ("error out"), "mode (read-only)"=H5Fmode."read-write", "path"=w479) -> ("error out"=w477:errorcluster, "ref out"=w476:T10)  [unwired: 7 in]
                                n200 = global read "Global.vi" "SQUID"() -> (w470:string)
                                n201 = call <vilib>:"H5Gopen.vi"("create? (F)"=TRUE, "error in (no error)"=w477, "name"=w470, "ref in"=w476) -> ("error out"=w472:errorcluster, "group out"=w473:T10)  [unwired: 6 in]
                                n202 = xnode "H5Awrite.xnode"("error in (no error)"=w472, "data"=w474, "attrib name"="DATETIME", "ref in"=w473) -> ("error out"=w460:errorcluster, "ref out"=w461:i32)  [unwired: 3 in, 1 out]
                                n203 = xnode "H5Awrite.xnode"("error in (no error)"=w460, "data"=w468, "attrib name"="LOOP", "ref in"=w461) -> ("error out"=w467:errorcluster, "ref out"=w464:i32)  [unwired: 3 in, 1 out]
                                n204 = xnode "H5Awrite.xnode"("error in (no error)"=w467, "data"=w462, "attrib name"="SQUID", "ref in"=w464) -> ("error out"=w466:errorcluster, "ref out"=w465:i32)  [unwired: 3 in, 1 out]
                                n205 = call <vilib>:"H5Gclose.vi"("error in (no error)"=w466, "group in"=w465) -> ("error out"=w475:errorcluster)  [unwired: 9 in]
                                n206 = call <vilib>:"H5Fclose.vi"("error in (no error)"=w475, "ref"=w476) -> ("error out"=w458:errorcluster)  [unwired: 9 in]
                                n207 = local write "hdf5"(w458) -> ()
                                n208 = call "error_log.vi"("error"=w458) -> ()  [unwired: 10 in]
                                }
                              }
                            }
                          }
                        }
                        n209 = call <vilib>:"Release Semaphore.vi"("error in (no error)"=w366, "semaphore"=w368) -> ("error out"=w370:errorcluster, "semaphore out"=w369:T9)  [unwired: 4 in]
                        n210 = call <vilib>:"Release Semaphore Reference.vi"("error in (no error)"=w370, "semaphore"=w369) -> ()  [unwired: 8 in, 2 out]
                      }
                      frame #2 {
                        # "[2.2] acquire data"
                        n211 = flat-sequence {
                          tunnel: [w549] -> w535
                          frame #0 {
                            w549 = variant ("data")
                            # "Clear metadata\n record."
                            n212 = global write "Global.vi" "Rec"(w549) -> ()
                          }
                        }
                        n213 = local read "Loops"() -> (w541:i32)
                        n214 = local read "Lines"() -> (w542:i32)
                        n215 = Get Date/Time In Seconds() -> (seconds since 1Jan1904=w539:timestamp)
                        n216 = local read "Abort"() -> (w546:bool)
                        n217 = To Double Precision Float(number=w539) -> (double precision float=w538:dbl)
                        n218 = Multiply(x=w542, y=w541) -> (x*y=w540:i32)
                        n219 = case shown="False" w546 {
                          selector: w546 -> [_ w745]
                          tunnel: w548 -> [w704 w746]
                          tunnel: [w708 w746] -> w544
                          tunnel: [w706 w745] -> w547
                          tunnel: w540 -> [w705 _]
                          tunnel: [w703 w744] -> w537
                          tunnel: w538 -> [w701 w744]
                          tunnel: [w699 w744] -> w536
                          tunnel: w535 -> [_ _]
                          frame False {
                            n220 = flat-sequence {
                              tunnel: [w712] -> w710
                              tunnel: w705 -> [w711]
                              tunnel: w701 -> [w712]
                              tunnel: [w723] -> w709
                              tunnel: w710 -> [w720]
                              tunnel: [w724] -> w707
                              tunnel: w704 -> [w721]
                              tunnel: [w720] -> w702
                              tunnel: [w719] -> w700
                              tunnel: [w743] -> w708
                              tunnel: w709 -> [w743]
                              tunnel: w707 -> [w741]
                              tunnel: [w741] -> w706
                              tunnel: [w740] -> w703
                              tunnel: w702 -> [w740]
                              tunnel: [w739] -> w699
                              tunnel: w700 -> [w739]
                              frame #0 {
                                n221 = global read "Global.vi" "SQUID"() -> (w713:string)
                                n222 = Number To Decimal String(number=w711) -> (decimal integer string=w716:string)  [unwired: 1 in]
                                n223 = global write "Global.vi" "Acquire"(TRUE ("Save")) -> ()
                                n224 = Concatenate Strings("Running " ("Status"), w713, " of " ("string"), w716) -> (w715:string)
                                n225 = local write "Status"(w715) -> ()
                              }
                              frame #1 {
                                # "Acquire data."
                                n226 = while {
                                tunnel: w720 -> [w736]
                                tunnel: [FALSE ("Save")] -> w722
                                tunnel: [w725] -> w724
                                shift-right: [w732] -> w723
                                shift-left: w721 -> [w732]
                                tunnel: [w726] -> w719
                                stop <- w733 stop-if-true
                                n227 = Get Date/Time In Seconds() -> (seconds since 1Jan1904=w737:timestamp)
                                n228 = Wait (ms)(milliseconds to wait=u32 200) -> ()  [unwired: 1 out]
                                n229 = To Double Precision Float(number=w737) -> (double precision float=w726:dbl)
                                n230 = Subtract(x=w726, y=w736) -> (x-y=w729:dbl)
                                n231 = To Double Precision Float(number="Acquire (s)") -> (double precision float=w727:dbl)
                                n232 = To Long Integer(number=w729) -> (32bit integer=→"Elapsed (s)":i32)
                                n233 = local read "Abort"() -> (w725:bool)
                                n234 = Greater Or Equal?(x=w729, y=w727) -> (x >= y?=w734:bool)
                                n235 = global read "Global.vi" "EOS"() -> (w730:bool)
                                n236 = Compound Arithmetic op=OR(w730, w734, w725) -> (w733:bool)
                                }
                                n237 = global write "Global.vi" "EOS"(w722) -> ()
                                n238 = global write "Global.vi" "Acquire"(w722) -> ()
                              }
                              frame #2 {
                                n239 = local write "Status"("Done!" ("Status")) -> ()
                              }
                            }
                          }
                          frame True {
                          }
                        }
                        n240 = Unbundle By Name(w544) -> ("code"=w543:i32)
                        n241 = local write "error out"(w544) -> ()
                        n242 = case shown="True" w545 {
                          tunnel: w536 -> [_ w553]
                          tunnel: w543 -> [_ w552]
                          tunnel: w537 -> [_ w551]
                          frame False {
                          }
                          frame True {
                            n243 = call <vilib>:"Obtain Semaphore Reference.vi"("error in (no error)"=errorcluster {"status"=FALSE, "code"=0, "source"=""}, "name (unnamed)"="hdf5") -> ("error out"=w562:errorcluster, "semaphore"=w563:T9)  [unwired: 3 in, 1 out]
                            n244 = global read "Global.vi" "H5"() -> (w554:path[])
                            n245 = call <vilib>:"Acquire Semaphore.vi"("error in (no error)"=w562, "semaphore"=w563) -> ("error out"=w556:errorcluster, "semaphore out"=w555:T9)  [unwired: 3 in, 1 out]
                            n246 = for {
                              shift-right: [w600] -> w557
                              shift-left: w555 -> [w600]
                              shift-right: [w599] -> w558
                              shift-left: w556 -> [w599]
                              tunnel: w554 -> [w598] mode=indexing
                              tunnel: w553 -> [w569]
                              tunnel: w552 -> [w588]
                              tunnel: w551 -> [w568]
                              n247 = global read "Global.vi" "SQUID"() -> (w595:string)
                              n248 = call <vilib>:"H5Fopen.vi"("error in (no error)"=errorcluster {"status"=FALSE, "code"=0, "source"=""}, "mode (read-only)"=H5Fmode."read-write", "path"=w598) -> ("error out"=w596:errorcluster, "ref out"=w593:T10)  [unwired: 7 in]
                              n249 = call <vilib>:"H5Gopen.vi"("error in (no error)"=w596, "name"=w595, "ref in"=w593) -> ("error out"=w591:errorcluster, "group out"=w590:T10)  [unwired: 7 in]
                              n250 = xnode "H5Awrite.xnode"("error in (no error)"=w591, "data"=w588, "attrib name"="ERROR", "ref in"=w590) -> ("error out"=w573:errorcluster, "ref out"=w572:i32)  [unwired: 3 in, 1 out]
                              n251 = xnode "H5Awrite.xnode"("error in (no error)"=w573, "data"=w568, "attrib name"="START", "ref in"=w572) -> ("error out"=w570:errorcluster, "ref out"=w571:i32)  [unwired: 3 in, 1 out]
                              n252 = Subtract(x=w569, y=w568) -> (x-y=w567:dbl)
                              n253 = xnode "H5Awrite.xnode"("error in (no error)"=w570, "data"=w569, "attrib name"="END" ("object name"), "ref in"=w571) -> ("error out"=w586:errorcluster, "ref out"=w583:i32)  [unwired: 3 in, 1 out]
                              n254 = Empty String/Path?(string/path="SQUID Comment") -> (empty?=w582:bool)
                              n255 = case shown="False" w582 {
                                tunnel: [w624 w643] -> w585
                                tunnel: [w623 w644] -> w584
                                tunnel: w586 -> [w622 w643]
                                tunnel: w583 -> [w621 w644]
                                tunnel: "Comment" ("attrib name") -> [w620 _]
                                tunnel: "SQUID Comment" -> [w619 _]
                                frame False {
                                n256 = xnode "H5Awrite.xnode"("error in (no error)"=w622, "data"=w619, "attrib name"=w620, "ref in"=w621) -> ("error out"=w624:errorcluster, "ref out"=w623:i32)  [unwired: 3 in, 1 out]
                                }
                                frame True {
                                }
                              }
                              n257 = xnode "H5Awrite.xnode"("error in (no error)"=w585, "data"=w567, "attrib name"="ACQUIRE" ("object name"), "ref in"=w584) -> ("error out"=w578:errorcluster, "ref out"=w577:i32)  [unwired: 3 in, 1 out]
                              n258 = global read "Global.vi" "Rec"() -> (w579:variant)
                              n259 = call <vilib>:"H5Awrite_multi.vi"("error in (no error)"=w578, "variant in"=w579, "name prefix (none)"="REC:", "ref in"=w577) -> ("error out"=w575:errorcluster, "ref out"=w576:T10)  [unwired: 6 in]
                              n260 = call <vilib>:"H5Gclose.vi"("error in (no error)"=w575, "group in"=w576) -> ("error out"=w594:errorcluster)  [unwired: 9 in]
                              n261 = call <vilib>:"H5Fclose.vi"("error in (no error)"=w594, "ref"=w593) -> ("error out"=w564:errorcluster)  [unwired: 9 in]
                              n262 = local write "hdf5"(w564) -> ()
                              n263 = call "error_log.vi"("error"=w564) -> ()  [unwired: 10 in]
                            }
                            n264 = call <vilib>:"Release Semaphore.vi"("error in (no error)"=w558, "semaphore"=w557) -> ("error out"=w559:errorcluster, "semaphore out"=w560:T9)  [unwired: 4 in]
                            n265 = call <vilib>:"Release Semaphore Reference.vi"("error in (no error)"=w559, "semaphore"=w560) -> ()  [unwired: 8 in, 2 out]
                          }
                        }
                      }
                      frame #3 {
                        w748 = FALSE ("All Set")
                        # "[2.3] Reset"
                        n266 = local read "VARS"() -> (w749:T1)
                        n267 = for {
                          tunnel: [w752] -> w747 mode=indexing
                          tunnel: w749 -> [w750] mode=indexing
                          w751 = FALSE ("Set")
                          n268 = Bundle By Name(cluster=w750, "Recieved"=w751, "Recieved"=w751) -> (w752:T7)
                        }
                        n269 = local write "All Set"(w748) -> ()
                        n270 = local write "Send"(w748) -> ()
                        n271 = local write "Recieved"(w748) -> ()
                        n272 = local write "VARS"(w747) -> ()
                      }
                    }
                    n273 = local write "SQUID Comment"(w178) -> ()
                    n274 = Wait (ms)(milliseconds to wait=u32 2000) -> ()  [unwired: 1 out]
                  }
                  n275 = call "SEQ_to_VAR_str.vi"("SEQs IN"=w162) -> ("VAR Strings"=w163:string[])  [unwired: 9 in, 1 out]
                  n276 = local write "VAR string"(w163) -> ()
                  n277 = Greater Or Equal?(x=w161, y=w158) -> (x >= y?=w160:bool)
                  n278 = Or(x=w160, y=w157) -> (x .or. y?=w159:bool)
                }
              }
              frame #3 {
                # "[3] tidy up"
                n279 = flat-sequence {
                  frame #0 {
                    n280 = Wait (ms)(milliseconds to wait=u32 100) -> ()  [unwired: 1 out]
                  }
                  frame #1 {
                    w773 = T4."Enabled" ("Disabled")
                    w772 = FALSE ("Abort")
                    n281 = global write "Global.vi" "RID"("") -> ()
                    n282 = local write "Status"("<<Idle>>" ("Status")) -> ()
                    n283 = property on="stop" class="Bool"("DisabledEnum"=w773) -> ()  [unwired: 2 in, 2 out]
                    n284 = property on="Run" class="Bool"("DisabledEnum"=w773) -> ()  [unwired: 2 in, 2 out]
                    n285 = property on="Abort" class="Bool (strict)"("DisabledEnum"=T4."Disabled and Grayed Out" ("Disabled"), "Value"=w772) -> ()  [unwired: 2 in, 2 out]
                    n286 = property on="Save" class="Bool (strict)"("DisabledEnum"=w773) -> ()  [unwired: 2 in, 2 out]
                    n287 = property on="Load List" class="Bool"("DisabledEnum"=w773) -> ()  [unwired: 2 in, 2 out]
                    n288 = property on="SEQ File" class="Path"("DisabledEnum"=w773) -> ()  [unwired: 2 in, 2 out]
                    n289 = global write "Global.vi" "SEQLine"("END" ("Seq")) -> ()
                    n290 = global write "Global.vi" "Acquire"(w772) -> ()
                    n291 = global write "Global.vi" "Run"(w772) -> ()
                  }
                }
                n292 = case shown="False" w760 {
                  tunnel: ["###### End     RUN: " ("string") "###### Abort  RUN: " ("string")] -> w762
                  frame False {
                  }
                  frame True {
                  }
                }
                n293 = local read "RID"() -> (w766:string)
                n294 = flat-sequence {
                  tunnel: w761 -> [_]
                  frame #0 {
                    n295 = To Unsigned Long Integer(number=inf) -> (unsigned 32bit integer=w768:u32)
                    n296 = property on="Run List" class="Str"("Text.Scroll Position"=w768) -> ()  [unwired: 2 in, 2 out]
                  }
                }
                n297 = local read "Run List"() -> (w764:string)
                n298 = Concatenate Strings(w762, w766, " ######" ("string")) -> (w756:string)
                n299 = Concatenate Strings(w764, w756, "\r") -> (w761:string)
                n300 = local write "Run List"(w761) -> ()
                n301 = Get Date/Time In Seconds() -> (seconds since 1Jan1904=w757:timestamp)
                n302 = Bundle("seconds since 1Jan1904"=w757, w756) -> (w755:T2)  [unwired: 1 in]
                n303 = Send Notification(notification=w755, notifier=w758, error in (no error)=w759) -> (notifier out=w754:refnum<notifier>, error out=w753:errorcluster)
              }
            }
          }
          event "SEQ File": Mouse Wheel {
            # "scroll through previous osq files"
            n304 = event-data() -> ("Delta"=w789:i32)  [unwired: 1 in, 9 out]
            n305 = local read "uFiles"() -> (w787:path[])
            n306 = Array Size(array=w787) -> (size(s)=w784:i32)
            n307 = feedback #1(0 ("f")) -> (w782:i32)
            n308 = Add(x=w789, y=w782) -> (x+y=w788:i32)
            n309 = Decrement(x=w784) -> (x-1=w783:i32)
            n310 = In Range and Coerce(upper limit=w783, x=w788, lower limit=0 ("f")) -> (coerced(x)=w781:i32)  [unwired: 1 out]
            n311 = feedback-in #1(w781) -> ()
            n312 = Index Array(array=w787, index=w781) -> (element=w786:path)
            n313 = local write "SEQ File"(w786) -> ()
          }
          event "Save": Value Change {
            n314 = event-data() -> ()  [unwired: 1 in, 5 out]
            n315 = case shown="True" "Save" {
              tunnel: [u32 14417920 u32 0] -> w792
              frame False {
              }
              frame True {
              }
            }
            n316 = property on="Run List" class="Str"("Text.BGColor"=w792) -> ()  [unwired: 2 in, 2 out]
          }
          event "Load List", "SEQ File": Value Change {
            n317 = event-data() -> ()  [unwired: 1 in, 6 out]
            n318 = local read "SEQ File"() -> (w801:path)
            n319 = Empty String/Path?(string/path=w801) -> (empty?=w800:bool)
            n320 = case shown="False" w800 {
              tunnel: w801 -> [w804 _]
              tunnel: [w805 string[] [] ("VAR string")] -> w798
              tunnel: [w802 0 ("Total Lines")] -> w799
              frame False {
                n321 = call "OSQ_load.vi"("Open"=w804) -> ("SEQs"=w803:T5[], "Lines"=w802:i32)  [unwired: 7 in, 2 out]
                n322 = call "SEQ_to_VAR_str.vi"("SEQs IN"=w803) -> ("VAR Strings"=w805:string[])  [unwired: 9 in, 1 out]
              }
              frame True {
              }
            }
            n323 = local write "VAR string"(w798) -> ()
            n324 = local write "Lines"(w799) -> ()
          }
          event "stop": Value Change {
            n325 = event-data() -> ()  [unwired: 1 in, 5 out]
          }
        }
      }
    }
  }
  n326 = Release Notifier(notifier=w2, error in (no error)=w3) -> (error out=w1:errorcluster)  [unwired: 1 in, 2 out]
  n327 = call <vilib>:"Simple Error Handler.vi"("error in (no error)"=w1) -> ()  [unwired: 4 in, 5 out]
